vi "PicoScope5000aUnitInfo.vi"(4 "handle in":i16, 5 "error in (no error)":errorcluster) -> (0 "Unit Info":T1, 1 "handle out":i16, 2 "error out":errorcluster)   [LabVIEW 2020]
uses:
  ps5000a.dll
panel:
  out "PICO_STATUS":u32
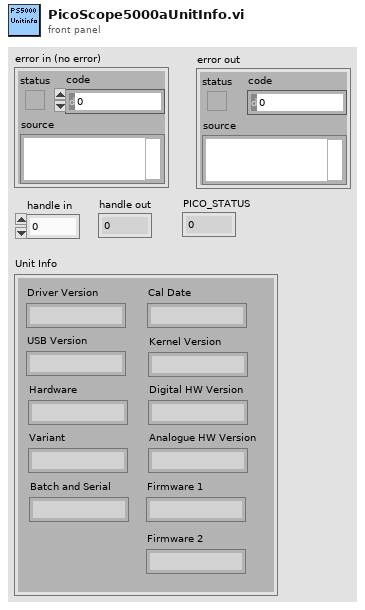
[diagram p1: front panel]
types:
  T1 = cluster{"Driver Version":string, "USB Version":string, "Hardware":string, "Variant":string, "Batch and Serial":string, "Cal Date":string, "Kernel Version":string, "Digital HW Version":string, "Analogue HW Version":string, "Firmware 1":string, "Firmware 2":string}
  T2 = cluster{"[0]":string, "[1]":string, "[2]":string, "[3]":string, "[4]":string, "[5]":string, "[6]":string, "[7]":string, "[8]":string, "[9]":string, "[10]":string}
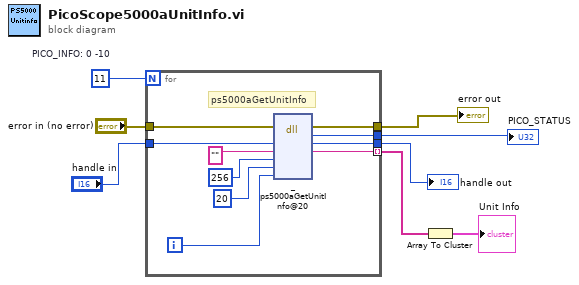
[diagram p0: block diagram]
diagram:
  w7 = 11  # PICO_INFO: 0 -10
  n1 = for {
    N: w7 -> [_]
    tunnel: "handle in" -> [w18]
    tunnel: [w15] -> w3 mode=indexing
    tunnel: "error in (no error)" -> [w12]
    tunnel: [w11] -> w5
    tunnel: [w10] -> w1
    tunnel: [w9] -> w4
    i -> [w13]
    # "ps5000aGetUnitInfo"
    n2 = dll-call lib="ps5000a.dll" fn="_ps5000aGetUnitInfo@20"(error in=w12, "handle"=w18, "unitInfo"="", "stringLength"=i16 256, "requiredSize"=i16 20 ("stringLength"), "pico_info"=w13) -> (error out=w10:errorcluster, "PICO_STATUS"=w9:u32, "handle"=w11:i16, "unitInfo"=w15:string)  [unwired: 5 in, 1 out]
  }
  "error out" <- w1
  "handle out" <- w5
  "PICO_STATUS" <- w4
  n3 = Array To Cluster(array=w3) -> (cluster=→"Unit Info":T2)
